vi "例7-5(1).vi"() -> ()   [LabVIEW 2019]
panel:
  out "告警":bool
  out "闸门开启高度(m)":dbl=9.58 format="%_3g"
  out "水流量(m^3/s)":dbl=5.927 format="%_4g"
  out "水位(m)":dbl=22.25 format="%#_4g"
  in  "写入位置":string="dstp://localhost/water"
  in  "停止按钮":bool
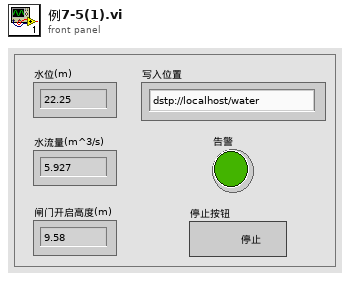
[diagram p1: front panel]
types:
  T1 = enum16{"Read", "Write", "ReadWrite", "BufferedRead", "BufferedReadWrite"}
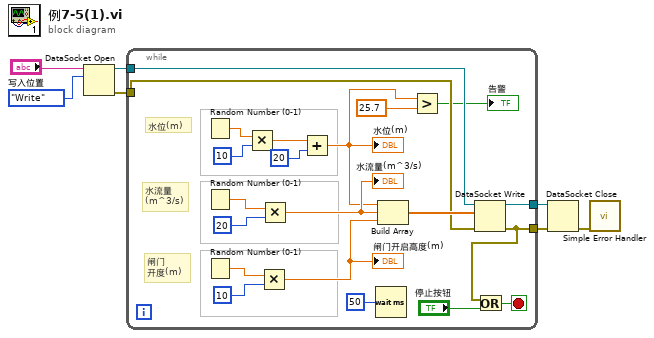
[diagram p0: block diagram]
diagram:
  n1 = DataSocket Open(10:T1."Write" ("模式"), 11:"写入位置") -> (0:w4:errorcluster, 3:w5:refnum<k13>)  [unwired: 2 in]
  n2 = while {
    tunnel: [w18] -> w3
    tunnel: w5 -> [w15]
    tunnel: w4 -> [w12]
    tunnel: [w11] -> w1
    stop <- w16 stop-if-true
    # "闸门\n开度(m)"
    # "水流量\n(m^3/s)"
    # "水位(m)"
    n3 = Random Number (0-1)() -> (number: 0 to 1=w28:dbl)
    n4 = Random Number (0-1)() -> (number: 0 to 1=w25:dbl)
    n5 = Random Number (0-1)() -> (number: 0 to 1=w21:dbl)
    n6 = Multiply(x=w28, y=10) -> (x*y=w26:dbl)
    n7 = Multiply(x=w21, y=10) -> (x*y=w13:dbl)
    "闸门开启高度(m)" <- w13
    n8 = Multiply(x=w25, y=20) -> (x*y=w14:dbl)
    "水流量(m^3/s)" <- w14
    n9 = Add(x=w26, y=20) -> (x+y=w10:dbl)
    "水位(m)" <- w10
    n10 = Wait (ms)(milliseconds to wait=50) -> ()  [unwired: 1 out]
    n11 = Build Array(w10, w14, w13) -> (w20:dbl[])
    n12 = Greater?(x=w10, y=25.7) -> (0:→"告警":bool)
    n13 = DataSocket Write(8:w12, 10:w20, 11:w15) -> (0:w18:errorcluster, 3:w11:refnum<k13>)  [unwired: 1 in, 1 out]
    n14 = Or(x=w18, y="停止按钮") -> (x .or. y?=w16:bool)
  }
  n15 = DataSocket Close(8:w3, 11:w1) -> (0:w2:errorcluster)  [unwired: 1 in, 1 out]
  n16 = call <vilib>:"Simple Error Handler.vi"("error in (no error)"=w2) -> ()  [unwired: 4 in, 5 out]
